vi "Delay Doubble.vi"(2 "Enum":T1(ring), 5 "input":dbl, 9 "Delay":i32) -> (6 "Output":dbl, 8 "Debounced":dbl, 10 "History":dbl[](array[numeric]))   [LabVIEW 2016]
doc: "Every milisecond this VI inserts the value of the input terminal into an array at an index equal to delay pushing every other value in the array one index toward zero. The output terminal is equal to the zero index of the array. The array can be retrived from the history terminal and the average of the array can be retrived from the debounced terminal.\n\nThe mode terminal sets the mode of the delay. when the mode is set to falling the VI reinitializes the entire array as true when the button is pressed. In falling mode it reintitializes it as false when the button is released. Neither mode will not reinitalize when the input changes. Instant mode will remove the milisecond wait and complete all of the tasks once per cycle.\n\nWhen the Value of the delay terminal is changed the array is reinitialized as false.\n\nWhen the boolean polymorphic subVI recives true on the invert terminal it inverts it's input and all array initializations/reinitializations.\n\nWhen the doubble or integer polymorphic subVI is set to falling mode it sends the input directly to the output until it is set to zero. when set to zero it will send the last non zero value for delay ms. Rising mode does the opposite. \n\nCreated by Team 4130 for use in the 2016-2017 FRC season"
uses:
  <vilib>/Analysis/baseanly.llb/Mean (DBL).vi
  <vilib>/Analysis/NI_AALBase.lvlib
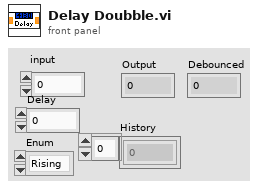
[diagram p1: front panel]
types:
  T1 = enum16{"Rising", "Falling", "Neither", "Instant"}
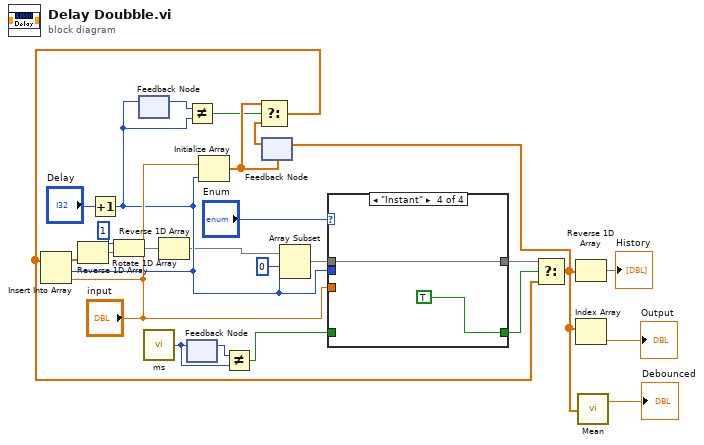
[diagram p0: block diagram]
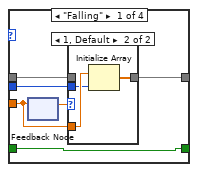
[diagram p2: hidden frame]
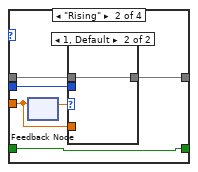
[diagram p4: hidden frame]
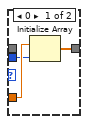
[diagram p5: hidden frame]
diagram:
  n1 = Increment(x="Delay") -> (x+1=w4:i32)
  n2 = feedback #1() -> (w8:i32)  [unwired: 1 in]
  n3 = feedback-in #1(w4) -> ()
  n4 = call "ms.vi"() -> ("millisecond"=w24:u32)  [unwired: 1 in]
  n5 = Not Equal?(x=w8, y=w4) -> (x != y?=w6:bool)
  n6 = feedback #2() -> (w25:u32)  [unwired: 1 in]
  n7 = feedback-in #2(w24) -> ()
  n8 = Initialize Array("input", w4) -> (w10:dbl[])
  n9 = Not Equal?(x=w25, y=w24) -> (x != y?=w15:bool)
  n10 = feedback #3(w10) -> (w9:dbl[])
  n11 = Select(t=w10, s=w6, f=w9) -> (s? t:f=w1:dbl[])
  n12 = Insert Into Array(array=w1, index=w4, new element="input") -> (w2:dbl[])
  n13 = Reverse 1D Array(array=w2) -> (reversed array=w21:dbl[])
  n14 = Rotate 1D Array(1:w21, 2:1 ("n")) -> (0:w23:dbl[])
  n15 = Reverse 1D Array(array=w23) -> (reversed array=w3:dbl[])
  n16 = Array Subset(array=w3, index=0, length=w4) -> (w14:dbl[])
  n17 = case shown="\"Instant\"" "Enum" {
    tunnel: w14 -> [w29 w39 w47 w49]
    tunnel: [w31 w41 w47 w49] -> w20
    tunnel: "input" -> [w28 w38 _ _]
    tunnel: w4 -> [w30 w40 _ _]
    tunnel: [w26 w36 w46 TRUE] -> w16
    tunnel: w15 -> [w26 w36 w46 _]
    frame "Falling" {
      n18 = feedback-in #4(w28) -> ()
      n19 = feedback #4() -> (w27:dbl)  [unwired: 1 in]
      n20 = case shown="1, Default" w27 {
        tunnel: [w32 w35] -> w31
        tunnel: w28 -> [_ w34]
        tunnel: w30 -> [_ w33]
        tunnel: w29 -> [w32 _]
        frame 0 {
        }
        frame 1, Default {
          n21 = Initialize Array(w34, w33) -> (w35:dbl[])
        }
      }
    }
    frame "Rising" {
      n22 = feedback-in #5(w38) -> ()
      n23 = feedback #5() -> (w37:dbl)  [unwired: 1 in]
      n24 = case shown="1, Default" w37 {
        tunnel: [w44 w45] -> w41
        tunnel: w38 -> [w43 _]
        tunnel: w40 -> [w42 _]
        tunnel: w39 -> [_ w45]
        frame 0 {
          n25 = Initialize Array(w43, w42) -> (w44:dbl[])
        }
        frame 1, Default {
        }
      }
    }
    frame "Neither", Default {
    }
    frame "Instant" {
    }
  }
  n26 = Select(t=w20, s=w16, f=w1) -> (s? t:f=w12:dbl[])
  n27 = feedback-in #3(w12) -> ()
  n28 = Reverse 1D Array(array=w12) -> (reversed array=→"History":dbl[])
  n29 = Index Array(array=w12) -> (element=→"Output":dbl)  [unwired: 1 in]
  n30 = call-poly <vilib>:"Mean.vi"("X"=w12) -> ("mean"=→"Debounced":dbl)  [unwired: 1 out]
